vi "P3-1.vi"() -> ()   [LabVIEW 2011]
panel:
  out "X/Y":dbl
  out "X*Y":dbl
  out "X-Y":dbl
  out "X+Y":dbl
  in  "Y":dbl(knob) scale=0.0..10.0
  in  "X":dbl(knob) scale=0.0..10.0
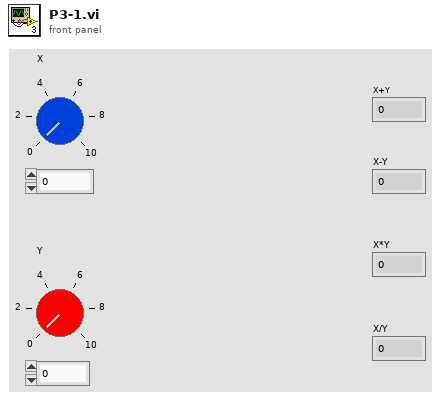
[diagram p1: front panel]
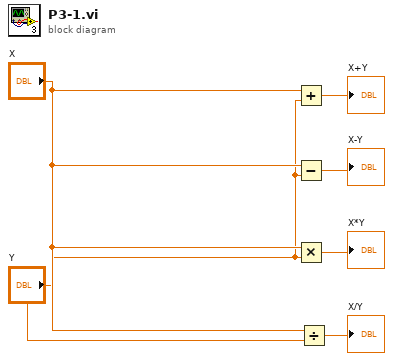
[diagram p0: block diagram]
diagram:
  n1 = Add(x="X", y="Y") -> (x+y=→"X+Y":dbl)
  n2 = Subtract(x="X", y="Y") -> (x-y=→"X-Y":dbl)
  n3 = Multiply(x="X", y="Y") -> (x*y=→"X*Y":dbl)
  n4 = Divide(x="X", y="Y") -> (x/y=→"X/Y":dbl)
